vi "Interface.vi"() -> ()   [LabVIEW 2016, in "Operation Interface.lvclass"]
uses:
  Operation Interface.lvclass
  Universal Robot/Universal Robot.lvclass
  C:/_Code/Development/UR LabVIEW Interface/Classes/Application Interface/Application Interface.lvclass
  Operation Interface.lvclass/Operation Interface.ctl
  Application Interface/RobotStatusFGV.ctl
  Application/Application.lvclass
  Application Interface/Application Interface.lvclass
panel:
  out "robotMode":string
  out "robotModeColor":u32(colorbox)
  out "operationalMode":string
  in  "powerOn":bool
  in  "brakeRelease":bool
  out "safetyStatus":string
  out "safetyStatusColor":u32(colorbox)
  in  "restartSafety":bool
  in  "unlockProtectiveStop":bool
  in  "shutdownRobot":bool
  in  "interface":refnum<class "Operation Interface.lvclass">
  in  "robot":refnum<class "Universal Robot.lvclass">
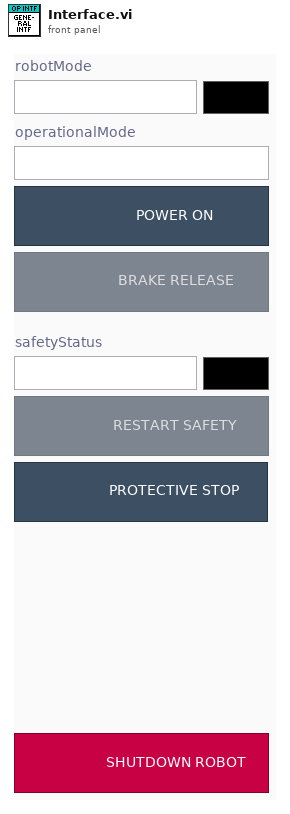
[diagram p1: front panel]
types:
  T1 = typedef "Application Interface.lvclass/RobotStatusFGV.ctl" = enum16{"Initialize", "Get Last Status", "Update Status"}
  T2 = typedef "Application.lvclass/FrontPanelControls.ctl" = cluster{"General Interface":refnum<vi>, "Program Interface":refnum<vi>, "Command Interface":refnum<vi>}
  T3 = typedef "Universal Robot.lvclass/RobotStatus.ctl" = cluster{"Robot Mode":T4, "Operational Mode":T5, "Safety Status":T6, "Remote Control":bool}
  T4 = typedef "Universal Robot.lvclass/RobotMode.ctl" = enum16{"INVALID", "NO_CONTROLLER", "DISCONNECTED", "CONFIRM_SAFETY", "BOOTING", "POWER_OFF", "POWER_ON", "IDLE", "BACKDRIVE", "RUNNING"}
  T5 = typedef "Universal Robot.lvclass/OperationalMode.ctl" = enum16{"NONE", "MANUAL", "AUTOMATIC"}
  T6 = typedef "Universal Robot.lvclass/SafetyStatus.ctl" = enum16{"INVALID", "NORMAL", "REDUCED", "PROTECTIVE_STOP", "RECOVERY", "SAFEGAURD_STOP", "SYSTEM_EMERGENCY_STOP", "ROBOT_EMERGENCY_STOP", "VIOLATION", "FAULT", "AUTOMATIC_MODE_SAFEGAURD_STOP", "SYSTEM_THREE_POSITION_ENABLING_STOP"}
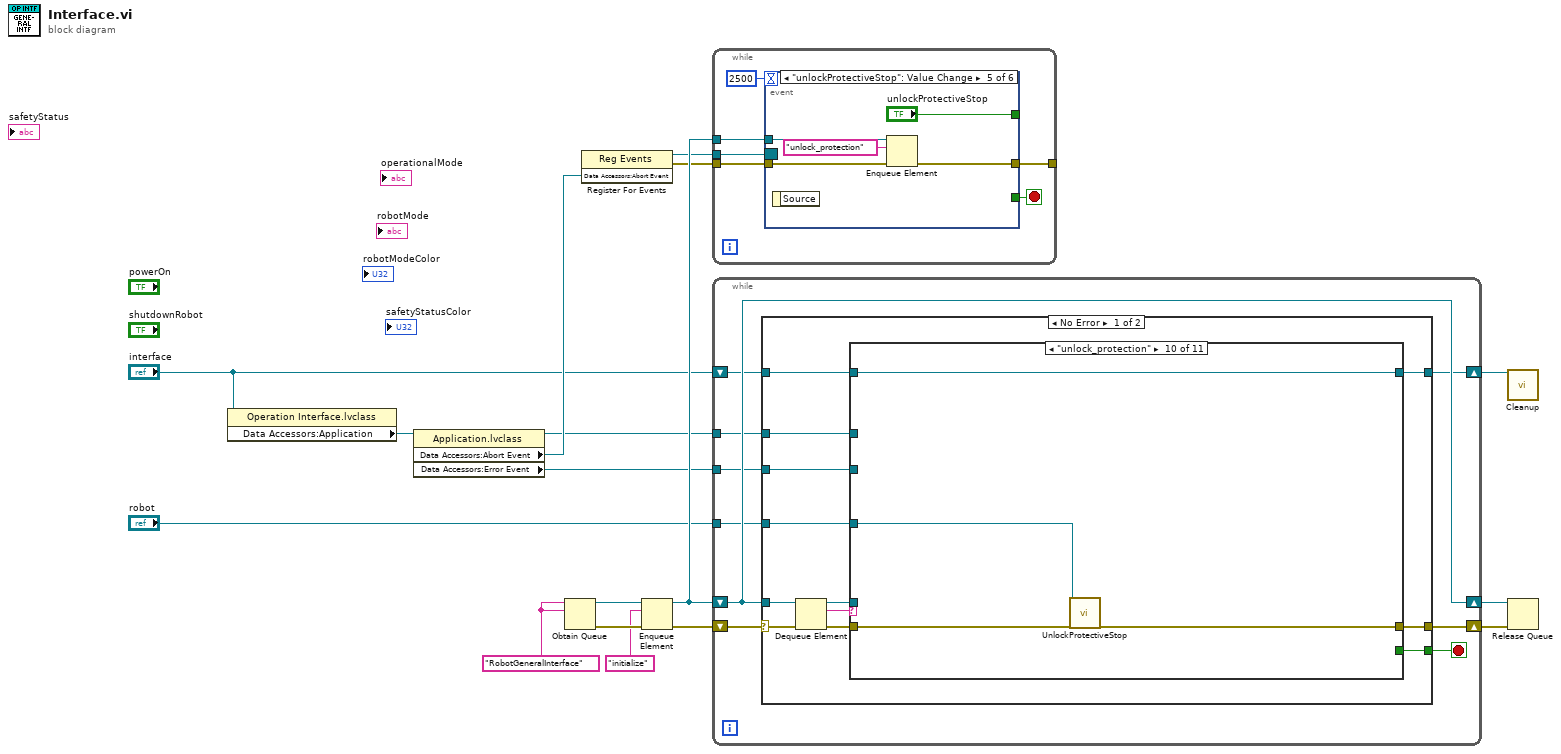
[diagram p0: block diagram]
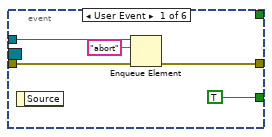
[diagram p2: hidden frame]
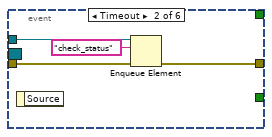
[diagram p3: hidden frame]
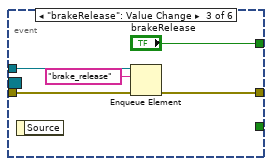
[diagram p4: hidden frame]
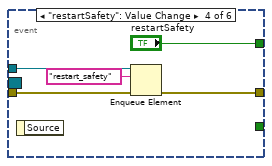
[diagram p5: hidden frame]
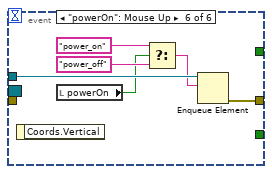
[diagram p6: hidden frame]
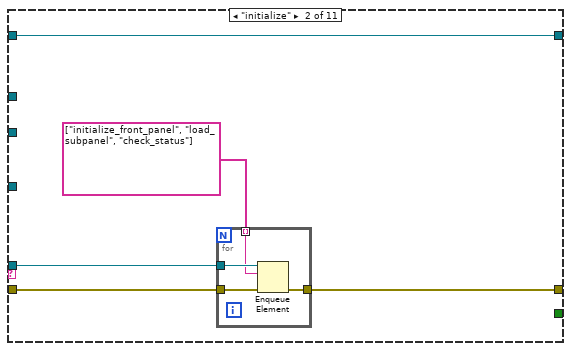
[diagram p8: hidden frame]
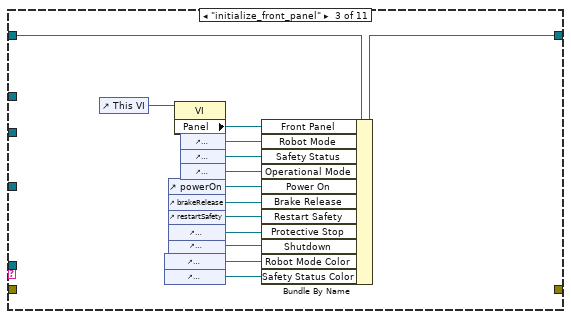
[diagram p9: hidden frame]
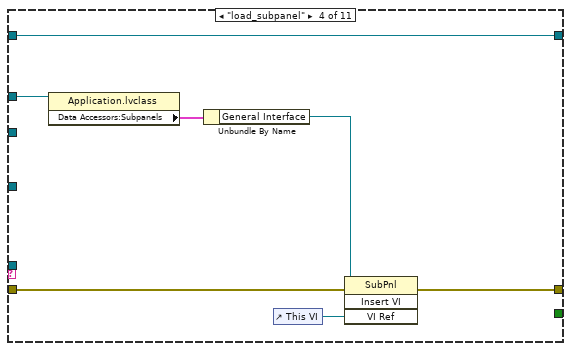
[diagram p10: hidden frame]
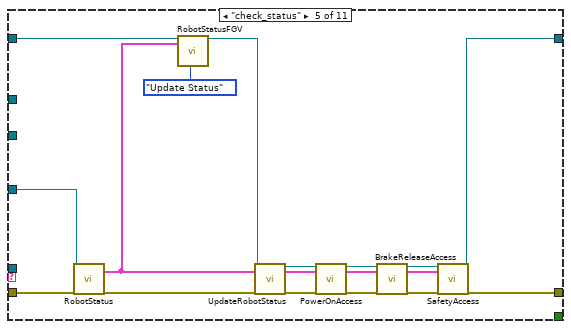
[diagram p11: hidden frame]
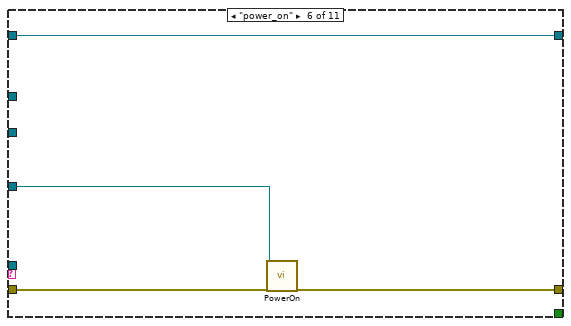
[diagram p12: hidden frame]
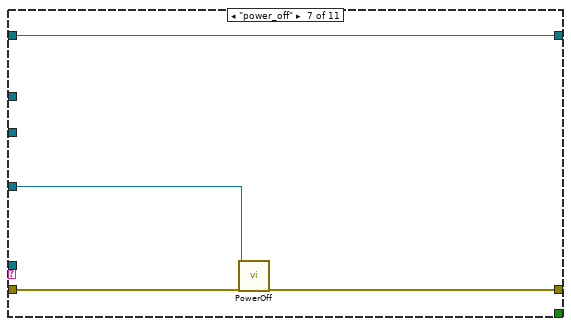
[diagram p13: hidden frame]
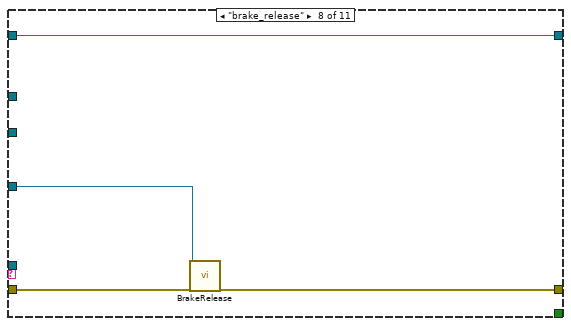
[diagram p14: hidden frame]
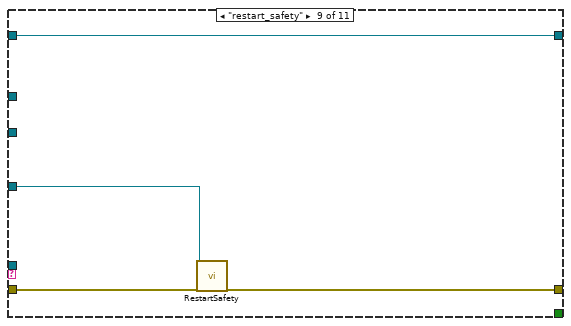
[diagram p15: hidden frame]
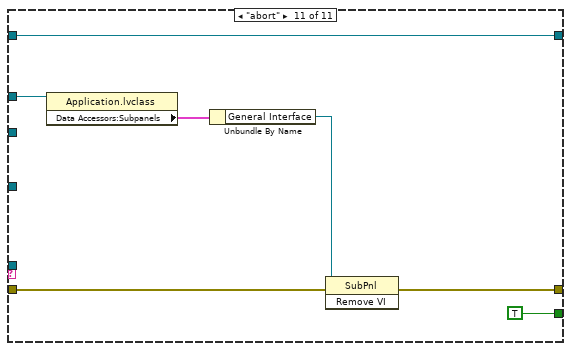
[diagram p16: hidden frame]
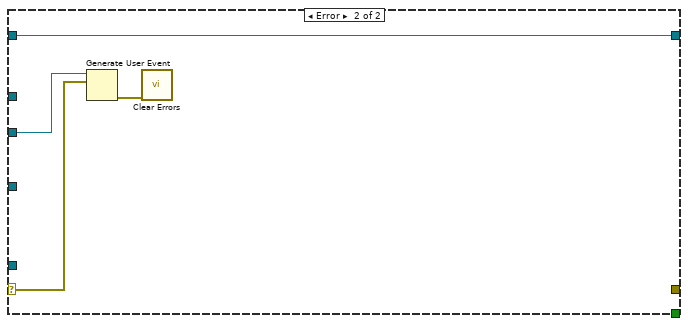
[diagram p17: hidden frame]
diagram:
  w12 = "RobotGeneralInterface" ("name (unnamed)")
  n1 = property class="Operation Interface.lvclass"(reference="interface") -> ("Data Accessors:Application"=w6:refnum<class "Application.lvclass">)  [unwired: 1 in, 2 out]
  n2 = property class="Application.lvclass"(reference=w6) -> (reference out=w3:refnum<class "Application.lvclass">, "Data Accessors:Abort Event"=w5:refnum<user-event>, "Data Accessors:Error Event"=w4:refnum<user-event>)  [unwired: 1 in, 1 out]
  n3 = Obtain Queue(name (unnamed)=w12, element data type=w12) -> (queue out=w16:refnum<queue>, error out=w17:errorcluster)  [unwired: 3 in, 1 out]
  n4 = register-events(w5) -> (reference out=w8:refnum<event-registration>, error out=w9:errorcluster)  [unwired: 2 in]
  n5 = Enqueue Element(queue=w16, element="initialize", error in (no error)=w17) -> (queue out=w13:refnum<queue>, error out=w14:errorcluster)  [unwired: 1 in, 1 out]
  n6 = while {
    tunnel: w13 -> [w23]
    tunnel: w9 -> [w22]
    tunnel: w8 -> [w21]
    tunnel: [w20] -> _
    stop <- w19 stop-if-true
    n7 = event shown="[4] \"unlockProtectiveStop\": Value Change" {
      selector: w21 -> [_ _ _ _ _ _]
      dyn-events: _ -> [_ _ _ _ _ _]
      timeout: 2500 -> [_ _ _ _ _ _]
      tunnel: w23 -> [w28 w32 w37 w42 w47 w53]
      tunnel: w22 -> [w27 w31 w36 w41 w46 _]
      tunnel: [w26 w30 w35 w40 w45 w52] -> w20
      tunnel: [TRUE _ _ _ _ _] -> w19
      tunnel: [_ _ "brakeRelease" "restartSafety" "unlockProtectiveStop" _] -> _
      event User Event {
        n8 = event-data() -> ()  [unwired: 1 in, 1 out]
        n9 = Enqueue Element(queue=w28, element="abort", error in (no error)=w27) -> (error out=w26:errorcluster)  [unwired: 1 in, 2 out]
      }
      event Timeout {
        n10 = event-data() -> ()  [unwired: 1 in, 1 out]
        n11 = Enqueue Element(queue=w32, element="check_status", error in (no error)=w31) -> (error out=w30:errorcluster)  [unwired: 1 in, 2 out]
      }
      event "brakeRelease": Value Change {
        n12 = event-data() -> ()  [unwired: 1 in, 1 out]
        n13 = Enqueue Element(queue=w37, element="brake_release", error in (no error)=w36) -> (error out=w35:errorcluster)  [unwired: 1 in, 2 out]
      }
      event "restartSafety": Value Change {
        n14 = event-data() -> ()  [unwired: 1 in, 1 out]
        n15 = Enqueue Element(queue=w42, element="restart_safety", error in (no error)=w41) -> (error out=w40:errorcluster)  [unwired: 1 in, 2 out]
      }
      event "unlockProtectiveStop": Value Change {
        n16 = event-data() -> ()  [unwired: 1 in, 1 out]
        n17 = Enqueue Element(queue=w47, element="unlock_protection", error in (no error)=w46) -> (error out=w45:errorcluster)  [unwired: 1 in, 2 out]
      }
      event "powerOn": Mouse Up {
        n18 = event-data() -> ()  [unwired: 1 in, 1 out]
        n19 = local read "powerOn"() -> (w48:bool)
        n20 = Select(t="power_on", s=w48, f="power_off") -> (s? t:f=w50:string)
        n21 = Enqueue Element(queue=w53, element=w50) -> (error out=w52:errorcluster)  [unwired: 2 in, 2 out]
      }
    }
  }
  n22 = while {
    shift-right: [w60] -> w10
    shift-left: w14 -> [w62]
    shift-right: [w61] -> w11
    shift-left: w13 -> [w61]
    tunnel: "robot" -> [w57]
    tunnel: w4 -> [w56]
    tunnel: w3 -> [w55]
    shift-right: [w54] -> w1
    shift-left: "interface" -> [w58]
    stop <- w59 stop-if-true
    n23 = case shown="No Error" w62 {
      selector: w62 -> [w73 w154]
      tunnel: w61 -> [w74 _]
      tunnel: [w69 _] -> w60
      tunnel: [w68 _] -> w59
      tunnel: w58 -> [w67 w152]
      tunnel: w57 -> [w66 _]
      tunnel: w56 -> [w65 w155]
      tunnel: w55 -> [w64 _]
      tunnel: [w63 w152] -> w54
      frame No Error {
        n24 = Dequeue Element(queue=w74, error in (no error)=w73) -> (queue out=w70:refnum<queue>, element=w71:string, error out=w72:errorcluster)  [unwired: 1 in, 1 out]
        n25 = case shown="\"unlock_protection\"" w71 {
          tunnel: w72 -> [w76 w79 _ w102 w124 w126 w131 w135 w139 w143 w149]
          tunnel: w70 -> [_ w80 _ _ _ _ _ _ _ _ _]
          tunnel: [w76 w78 _ w106 w109 w128 w129 w133 w137 w142 w148] -> w69
          tunnel: [_ _ _ _ _ _ _ _ _ _ TRUE] -> w68
          tunnel: w67 -> [w75 w81 w99 w104 w115 w125 w132 w136 w140 w144 w150]
          tunnel: w66 -> [_ _ _ _ w123 w127 w130 w134 w138 w141 _]
          tunnel: w65 -> [_ _ _ _ _ _ _ _ _ _ _]
          tunnel: w64 -> [_ _ _ w103 _ _ _ _ _ _ w147]
          tunnel: [w75 w81 w98 w104 w107 w125 w132 w136 w140 w144 w150] -> w63
          frame Default {
          }
          frame "initialize" {
            n26 = for {
              tunnel: w80 -> [w85]
              tunnel: w79 -> [w84]
              tunnel: [w83] -> w78
              tunnel: string[] ["initialize_front_panel", "load_subpanel", "check_status"] -> [w82] mode=indexing
              n27 = Enqueue Element(queue=w85, element=w82, error in (no error)=w84) -> (error out=w83:errorcluster)  [unwired: 1 in, 2 out]
            }
          }
          frame "initialize_front_panel" {
            n28 = control-ref of="This VI"() -> (w88:refnum<vi>)
            n29 = control-ref of="robotModeColor"() -> (w96:refnum<vi>)
            n30 = control-ref of="safetyStatusColor"() -> (w89:refnum<vi>)
            n31 = control-ref of="powerOn"() -> (w94:refnum<vi>)
            n32 = control-ref of="brakeRelease"() -> (w93:refnum<vi>)
            n33 = control-ref of="restartSafety"() -> (w92:refnum<vi>)
            n34 = control-ref of="unlockProtectiveStop"() -> (w91:refnum<vi>)
            n35 = control-ref of="shutdownRobot"() -> (w90:refnum<vi>)
            n36 = property class="VI"(reference=w88) -> ("Panel"=w87:refnum<vi>)  [unwired: 1 in, 2 out]
            n37 = control-ref of="robotMode"() -> (w97:refnum<vi>)
            n38 = control-ref of="safetyStatus"() -> (w86:refnum<vi>)
            n39 = control-ref of="operationalMode"() -> (w95:refnum<vi>)
            n40 = Bundle By Name(cluster=w99, "Front Panel"=w87, "Robot Mode"=w97, "Safety Status"=w86, "Operational Mode"=w95, "Power On"=w94, "Brake Release"=w93, "Restart Safety"=w92, "Protective Stop"=w91, "Shutdown"=w90, "Robot Mode Color"=w96, "Safety Status Color"=w89) -> (w98:refnum<class "Operation Interface.lvclass">)
          }
          frame "load_subpanel" {
            n41 = property class="Application.lvclass"(reference=w103) -> ("Data Accessors:Subpanels"=w101:T2)  [unwired: 1 in, 2 out]
            n42 = Unbundle By Name(w101) -> ("General Interface"=w100:refnum<vi>)
            n43 = control-ref of="This VI"() -> (w105:refnum<vi>)
            n44 = invoke class="SubPnl" method="Insert VI"(reference=w100, error in=w102, "VI Ref"=w105) -> (error out=w106:errorcluster)  [unwired: 1 in, 3 out]
          }
          frame "check_status" {
            n45 = call-dynamic "RobotStatus.vi"("Universal Robot.lvclass in"=w123, "error in (no error)"=w124) -> ("Robot Status"=w113:T3, "error out"=w122:errorcluster)  [unwired: 15 in, 1 out]
            n46 = call "RobotStatusFGV.vi"("Application Interface in"=w115, "Robot Status in"=w113, "Action (Read)"=RobotStatusFGV."Update Status") -> ("Application Interface out"=w114:refnum<class "Operation Interface.lvclass">)  [unwired: 14 in, 2 out]
            n47 = call "UpdateRobotStatus.vi"("Operation Interface in"=w114, "Robot Status"=w113, "error in (no error)"=w122) -> ("Operation Interface out"=w121:refnum<class "Operation Interface.lvclass">, "Robot Status Out"=w120:T3, "error out"=w119:errorcluster)  [unwired: 14 in]
            n48 = call "PowerOnAccess.vi"("Operation Interface in"=w121, "Robot Status"=w120, "error in (no error)"=w119) -> ("Operation Interface out"=w118:refnum<class "Operation Interface.lvclass">, "Robot Status Out"=w116:T3, "error out"=w117:errorcluster)  [unwired: 14 in]
            n49 = call "BrakeReleaseAccess.vi"("Operation Interface in"=w118, "Robot Status in"=w116, "error in (no error)"=w117) -> ("Operation Interface out"=w111:refnum<class "Operation Interface.lvclass">, "Robot Status out"=w108:T3, "error out"=w110:errorcluster)  [unwired: 14 in]
            n50 = call "SafetyAccess.vi"("Operation Interface in"=w111, "Robot Status"=w108, "error in (no error)"=w110) -> ("Operation Interface out"=w107:refnum<class "Operation Interface.lvclass">, "error out"=w109:errorcluster)  [unwired: 15 in]
          }
          frame "power_on" {
            n51 = call-dynamic "PowerOn.vi"("Universal Robot.lvclass in"=w127, "error in (no error)"=w126) -> ("error out"=w128:errorcluster)  [unwired: 16 in, 1 out]
          }
          frame "power_off" {
            n52 = call-dynamic "PowerOff.vi"("Universal Robot.lvclass in"=w130, "error in (no error)"=w131) -> ("error out"=w129:errorcluster)  [unwired: 16 in, 1 out]
          }
          frame "brake_release" {
            n53 = call-dynamic "BrakeRelease.vi"("Universal Robot.lvclass in"=w134, "error in (no error)"=w135) -> ("error out"=w133:errorcluster)  [unwired: 16 in, 1 out]
          }
          frame "restart_safety" {
            n54 = call-dynamic "RestartSafety.vi"("Universal Robot.lvclass in"=w138, "error in (no error)"=w139) -> ("error out"=w137:errorcluster)  [unwired: 16 in, 1 out]
          }
          frame "unlock_protection" {
            n55 = call-dynamic "UnlockProtectiveStop.vi"("Universal Robot.lvclass in"=w141, "error in (no error)"=w143) -> ("error out"=w142:errorcluster)  [unwired: 16 in, 1 out]
          }
          frame "abort" {
            n56 = property class="Application.lvclass"(reference=w147) -> ("Data Accessors:Subpanels"=w146:T2)  [unwired: 1 in, 2 out]
            n57 = Unbundle By Name(w146) -> ("General Interface"=w145:refnum<vi>)
            n58 = invoke class="SubPnl" method="Remove VI"(reference=w145, error in=w149) -> (error out=w148:errorcluster)  [unwired: 1 in, 2 out]
          }
        }
      }
      frame Error {
        n59 = Generate User Event(user event=w155, event data cluster=w154) -> (error out=w153:errorcluster)  [unwired: 2 in, 1 out]
        n60 = call <vilib>:"Clear Errors.vi"("error in (no error)"=w153) -> ()  [unwired: 5 in, 2 out]
      }
    }
  }
  n61 = call "Cleanup.vi"("Operation Interface in"=w1) -> ()  [unwired: 19 in]
  n62 = Release Queue(queue=w11, error in (no error)=w10) -> ()  [unwired: 1 in, 3 out]
